vi "__vna_read_save.vi"() -> ()   [LabVIEW 2013]
panel:
  in  "Tab Control 2":enum32{"Page 1", "Page 2"}(tab)
  in  "Power dBm":dbl=-25.0 caption="Power, dBm" format="%#.3f"
  in  "Start Freq (Hz)":dbl=3090000000.0 min=100000.0 max=20000000000.0 format="%^#.6e"
  in  "Stop Freq":dbl=400000000.0 caption="Stop Freq (Hz):" format="%^#.3e"
  in  "Bandwidth:":dbl=1.0 caption="Bandwidth (1 to 1e6 Hz):" format="%#.3f"
  in  "Points:":i32=201
  in  "Tab Control":enum32{"Page 1"}(tab)
  in  "Boolean":bool
  in  "Name":string="data_labview_vna_noise(1)_"
  out "Phase":cluster{dbl[], dbl[]}(graph)
  out "Lin Mag":cluster{dbl[], dbl[]}(graph)
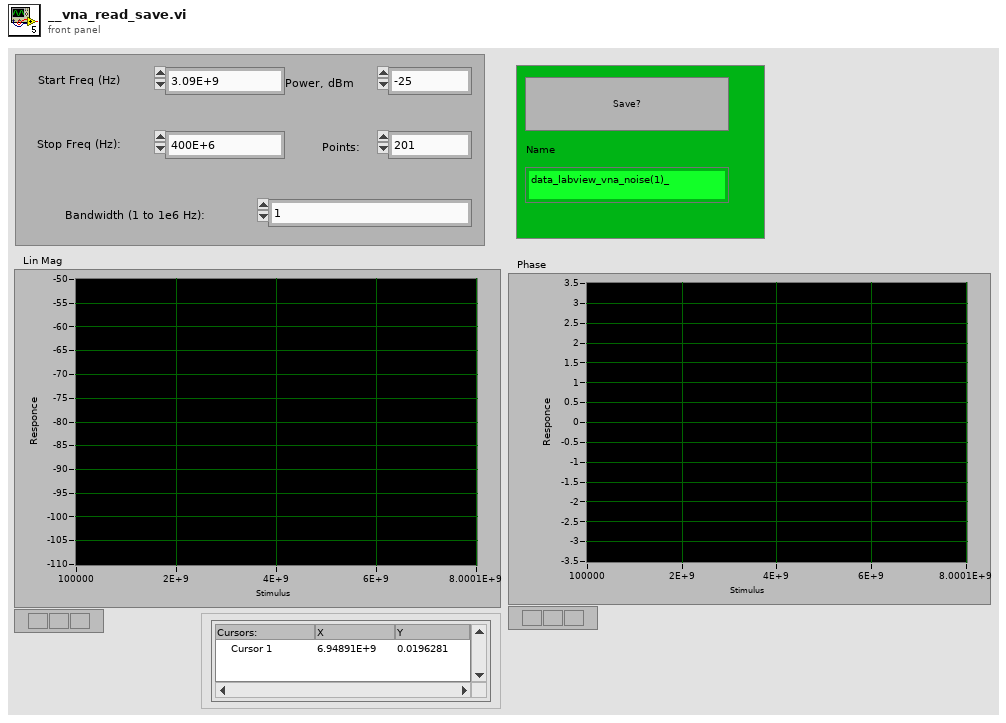
[diagram p1: front panel]
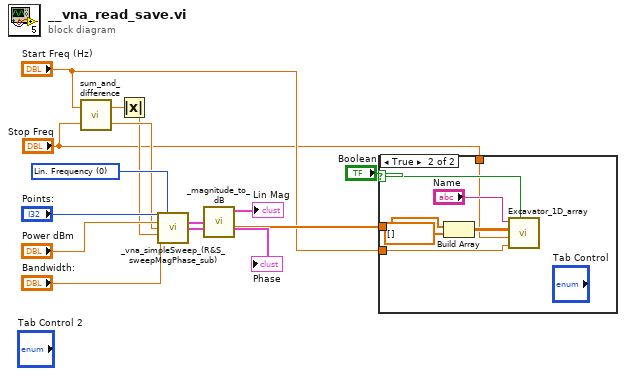
[diagram p0: block diagram]
diagram:
  w12 = 0 items=["Lin. Frequency", "Log. Frequency", "Segmented Frequency", "Power", "CW Mode", "Time"] ("Sweep Type")
  n1 = call "sum_and_difference.vi"("Begin"="Stop Freq", "End"="Start Freq (Hz)") -> ("Mid Point"=w4:dbl, "Difference (abs)"=w5:dbl)
  n2 = Absolute Value(x=w5) -> (abs(x)=w3:dbl)
  n3 = call "_vna_simpleSweep_(R&S_sweepMagPhase_sub).vi"("Sweep Type"=w12, "Points:"="Points:", "Power dBm"="Power dBm", "Center Freq:"=w4, "Span Freq:"=w3, "Bandwidth:"="Bandwidth:") -> ("Lin Mag"=w8:cluster{dbl[], dbl[]}, "Phase"=→"Phase":cluster{dbl[], dbl[]})  [unwired: 8 in]
  n4 = call "_magnitude_to_dB.vi"("Lin Mag in"=w8) -> ("Cluster"=→"Lin Mag":cluster{dbl[], dbl[]}, "dB"=w6:dbl[])  [unwired: 2 out]
  n5 = case shown="True" "Boolean" {
    selector: "Boolean" -> [_ w18]
    tunnel: w6 -> [_ w17]
    tunnel: "Start Freq (Hz)" -> [_ w16]
    tunnel: "Stop Freq" -> [_ w15]
    frame False {
    }
    frame True {
      n6 = Build Array(w17, dbl[] [] ("element")) -> (w20:dbl[][])
      n7 = call "Excavator_1D_array.vi"("Name"="Name", "Array"=w20, "x_max"=w15, "x_min"=w16, "Save?"=w18) -> ()  [unwired: 1 out]
    }
  }
